vi "Digital control.vi"(8 "error in":errorcluster, 10 "Digital I/O Pin (0)":u8=13, 11 "Arduino Resource":T1) -> (0 "error out":errorcluster, 3 "Arduino Resource out":T1={"VISA resource"="", "Board Type"=enum."Uno", "Connection Type"=enum."USB / Serial", "Bytes Per Packet (15)"=15})   [LabVIEW 2016]
uses:
  <vilib>/LabVIEW Interface for Arduino/Type Defs/Arduino Resource.ctl
  <vilib>/LabVIEW Interface for Arduino/Type Defs/Board Type.ctl
  <vilib>/LabVIEW Interface for Arduino/LabVIEW Interface for Arduino.lvlib
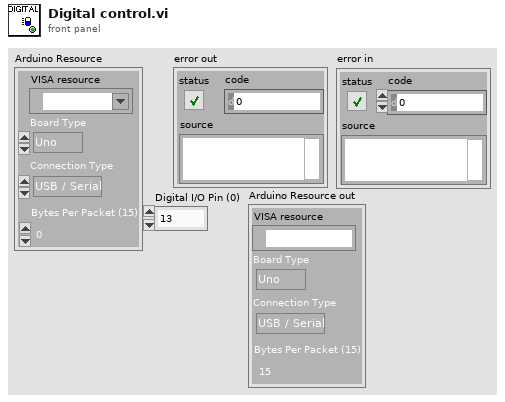
[diagram p1: front panel]
types:
  T1 = typedef "LabVIEW Interface for Arduino.lvlib/Arduino Resource.ctl" = cluster{"VISA resource":refnum<visa-resource-name>, "Board Type":T2, "Connection Type":enum8{"USB / Serial"}, "Bytes Per Packet (15)":u8}
  T2 = typedef "LabVIEW Interface for Arduino.lvlib/Board Type.ctl" = enum16{"Uno", "Dimuelanove w/Atmega 328", "Mega 2560"}
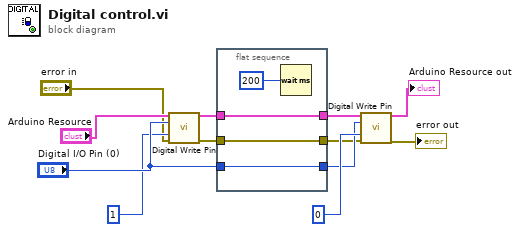
[diagram p0: block diagram]
diagram:
  n1 = call <vilib>:"Digital Write Pin.vi"("Arduino Resource"="Arduino Resource", "Digital I/O Pin (0)"="Digital I/O Pin (0)", "Value (0)"=u8 1, "error in"="error in") -> ("Arduino Resource"=w5:T1, "error out"=w6:errorcluster)  [unwired: 10 in]
  n2 = flat-sequence {
    tunnel: w5 -> [w15]
    tunnel: w6 -> [w14]
    tunnel: [w15] -> w7
    tunnel: [w14] -> w8
    tunnel: [w13] -> w9
    tunnel: "Digital I/O Pin (0)" -> [w13]
    frame #0 {
      n3 = Wait (ms)(milliseconds to wait=u32 200) -> ()  [unwired: 1 out]
    }
  }
  n4 = call <vilib>:"Digital Write Pin.vi"("Arduino Resource"=w7, "Digital I/O Pin (0)"=w9, "Value (0)"=u8 0, "error in"=w8) -> ("Arduino Resource"=→"Arduino Resource out":T1, "error out"=→"error out":errorcluster)  [unwired: 10 in]
